vi "FormatData.vi"(8 "ErrorIn":errorcluster, 11 "Packets":T1[](array[typedef])) -> (0 "ErrorOut":errorcluster, 3 "FormattedString":string)   [LabVIEW 2016]
doc: "Prepare text about important data in order to save it lately to a file."
uses:
  FallSensor/Packet.ctl
  FallSensor/Sample.ctl
  FallSensor/Reading.ctl
  FallSensor/ReadingUnits/AccelReadingUnit.ctl
  FallSensor/ReadingUnits/GyroReadingUnit.ctl
  FormatDataContext.ctl
  FileSection.ctl
panel:
  # "s"
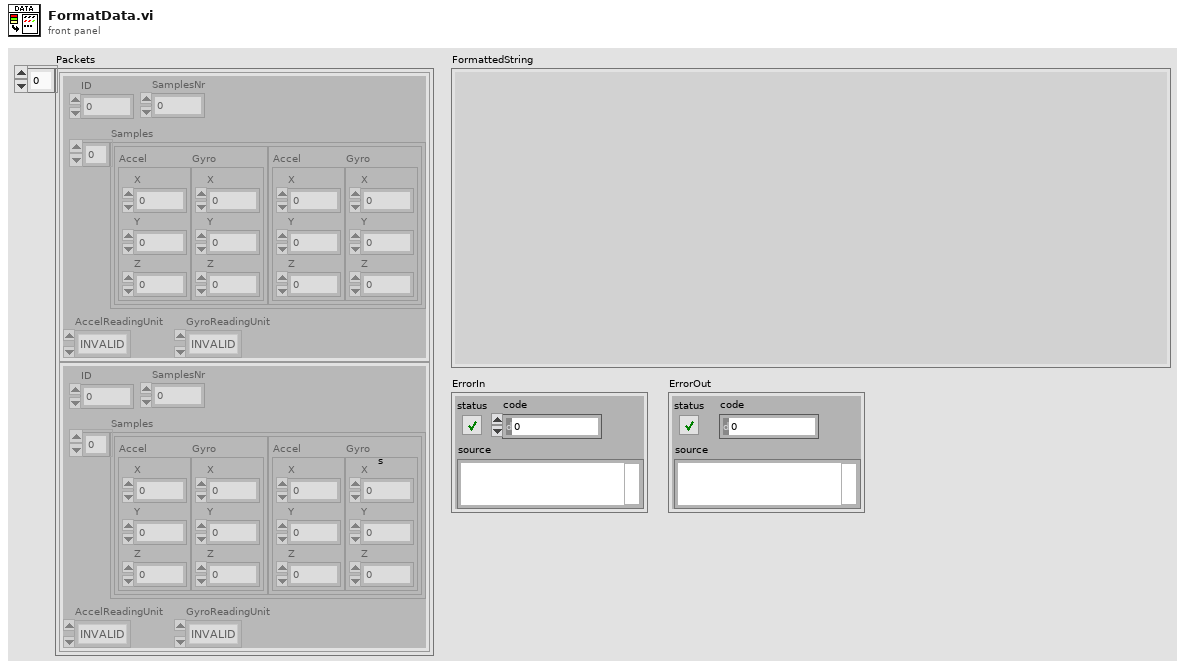
[diagram p1: front panel]
types:
  T1 = typedef "Packet.ctl" = cluster{"ID":u32, "SamplesNr":u32, "Samples":T2[], "AccelReadingUnit":T4, "GyroReadingUnit":T5}
  T2 = typedef "Sample.ctl" = cluster{"Accel":T3, "Gyro":T3}
  T3 = typedef "Reading.ctl" = cluster{"X":i16, "Y":i16, "Z":i16}
  T4 = typedef "AccelReadingUnit.ctl" = enum16{"INVALID", "RAW", "g"}
  T5 = typedef "GyroReadingUnit.ctl" = enum16{"INVALID", "RAW", "°/sec"}
  T6 = typedef "FileSection.ctl" = enum16{"SOF", "Header", "FileFormatVersion", "PacketsNumber", "Comment", "Data", "EOF"}
  T7 = typedef "FormatDataContext.ctl" = cluster{"Header":string, "FileFormatVersion":string, "Packets":T1[], "FormattedString":string}
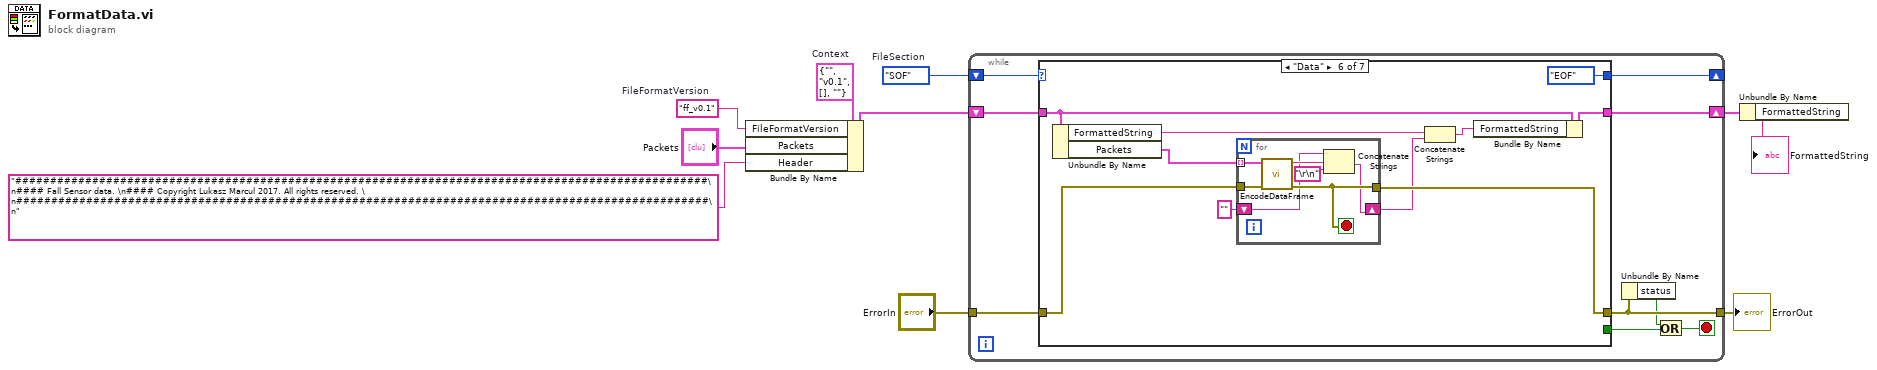
[diagram p0: block diagram]
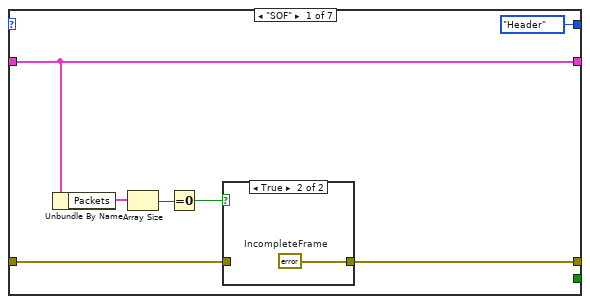
[diagram p2: hidden frame]
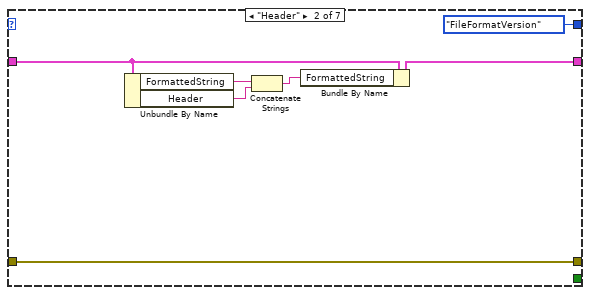
[diagram p4: hidden frame]
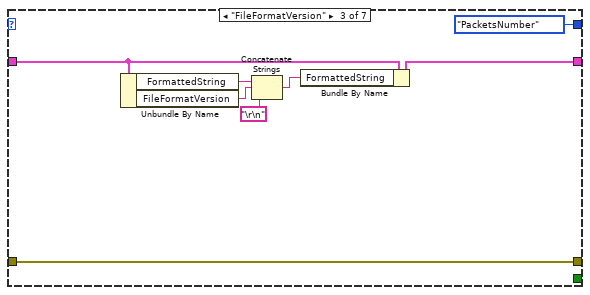
[diagram p5: hidden frame]
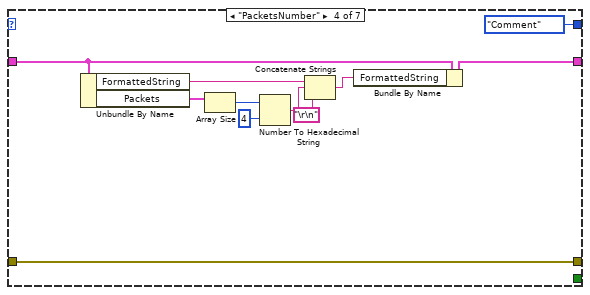
[diagram p6: hidden frame]
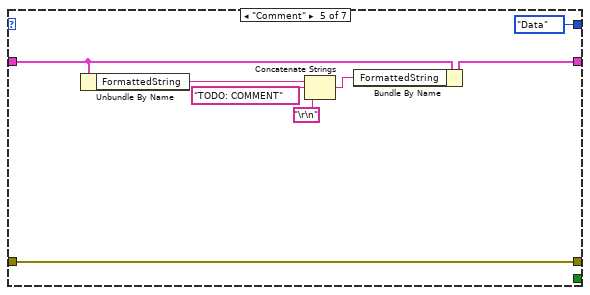
[diagram p7: hidden frame]
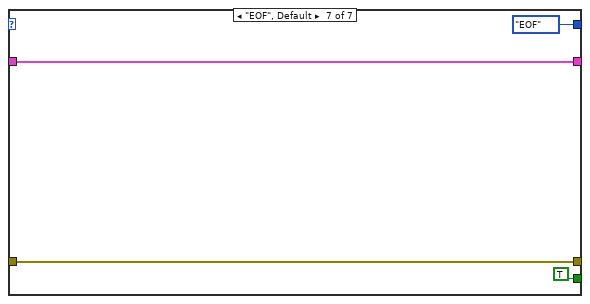
[diagram p8: hidden frame]
diagram:
  w7 = FileSection."SOF"  # FileSection
  w9 = "ff_v0.1"  # FileFormatVersion
  w10 = T7 {"Header"="", "FileFormatVersion"="v0.1", "Packets"=[], "FormattedString"=""}  # Context
  n1 = Bundle By Name(cluster=w10, "FileFormatVersion"=w9, "Packets"="Packets", "Header"="###################################################################################################\n#### Fall Sensor data. \n#### Copyright Lukasz Marcul 2017. All rights reserved. \n###################################################################################################\n") -> (w4:T7)
  n2 = while {
    tunnel: "ErrorIn" -> [w19]
    tunnel: [w14] -> w5
    shift-right: [w15] -> _
    shift-left: w7 -> [w18]
    shift-right: [w16] -> w2
    shift-left: w4 -> [w17]
    stop <- w12 stop-if-true
    n3 = case shown="\"Data\"" w18 {
      tunnel: w19 -> [w23 w30 w38 w50 w58 w65 w82]
      tunnel: [w22 w30 w38 w50 w58 w64 w82] -> w14
      tunnel: w17 -> [w20 w35 w43 w54 w62 w72 w83]
      tunnel: [w20 w31 w39 w51 w59 w69 w83] -> w16
      tunnel: [FileSection."Header" ("FileSection") FileSection."FileFormatVersion" ("FileSection") FileSection."PacketsNumber" ("FileSection") FileSection."Comment" ("FileSection") FileSection."Data" ("FileSection") FileSection."EOF" ("FileSection") FileSection."EOF" ("FileSection")] -> w15
      tunnel: [_ _ _ _ _ _ TRUE] -> w11
      frame "SOF" {
        n4 = Unbundle By Name(w20) -> ("Packets"=w26:T1[])
        n5 = Array Size(array=w26) -> (size(s)=w25:i32)
        n6 = Equal To 0?(x=w25) -> (x = 0?=w24:bool)
        n7 = case shown="True" w24 {
          tunnel: w23 -> [w27 _]
          tunnel: [w27 w28] -> w22
          frame False {
          }
          frame True {
            w28 = errorcluster {"status"=TRUE, "code"=1, "source"="Incomplete frame"}  # IncompleteFrame
          }
        }
      }
      frame "Header" {
        n8 = Unbundle By Name(w35) -> ("FormattedString"=w33:string, "Header"=w34:string)
        n9 = Concatenate Strings(w33, w34) -> (w32:string)
        n10 = Bundle By Name(cluster=w35, "FormattedString"=w32) -> (w31:T7)
      }
      frame "FileFormatVersion" {
        n11 = Unbundle By Name(w43) -> ("FormattedString"=w41:string, "FileFormatVersion"=w42:string)
        n12 = Concatenate Strings(w41, w42, "\r\n") -> (w40:string)
        n13 = Bundle By Name(cluster=w43, "FormattedString"=w40) -> (w39:T7)
      }
      frame "PacketsNumber" {
        n14 = Unbundle By Name(w54) -> ("FormattedString"=w53:string, "Packets"=w45:T1[])
        n15 = Array Size(array=w45) -> (size(s)=w46:i32)
        n16 = Number To Hexadecimal String(1:i16 4 ("width (-)"), 2:w46) -> (0:w48:string)
        n17 = Concatenate Strings(w53, w48, "\r\n") -> (w52:string)
        n18 = Bundle By Name(cluster=w54, "FormattedString"=w52) -> (w51:T7)
      }
      frame "Comment" {
        n19 = Unbundle By Name(w62) -> ("FormattedString"=w61:string)
        n20 = Concatenate Strings(w61, "TODO: COMMENT" ("string"), "\r\n") -> (w60:string)
        n21 = Bundle By Name(cluster=w62, "FormattedString"=w60) -> (w59:T7)
      }
      frame "Data" {
        n22 = Unbundle By Name(w72) -> ("FormattedString"=w71:string, "Packets"=w67:T1[])
        n23 = for {
          tunnel: w67 -> [w79] mode=indexing
          shift-right: [w73] -> w63
          shift-left: "" -> [w74]
          tunnel: w65 -> [w78]
          tunnel: [w77] -> w64
          stop <- w77 stop-if-true
          n24 = call "EncodeDataFrame.vi"("ErrorIn"=w78, "Packet"=w79) -> ("ErrorOut"=w77:errorcluster, "Frame"=w76:string)  [unwired: 8 in]
          n25 = Concatenate Strings(w74, w76, "\r\n") -> (w73:string)
        }
        n26 = Concatenate Strings(w71, w63) -> (w70:string)
        n27 = Bundle By Name(cluster=w72, "FormattedString"=w70) -> (w69:T7)
      }
      frame "EOF", Default {
      }
    }
    n28 = Unbundle By Name(w14) -> ("status"=w13:bool)
    n29 = Or(x=w13, y=w11) -> (x .or. y?=w12:bool)
  }
  "ErrorOut" <- w5
  n30 = Unbundle By Name(w2) -> ("FormattedString"=→"FormattedString":string)
